vi "LVClass_HasoEngine Set Preferences Multi Aperture.vi"(0 "HasoEngine in":refnum<class "HasoEngine.lvclass">, 5 "Start sub-aperture Array":T1[](array[typedef]), 7 "Pupil average":dbl=0.5 min=0.0 max=1.0, 9 "AutoStartSub-aperture":bool, 11 "error in (no error)":errorcluster) -> (4 "HasoEngine out":refnum<class "HasoEngine.lvclass">, 15 "error out":errorcluster)   [LabVIEW 2020, in "HasoEngine.lvclass"]
doc: "HasoSlopes computation preferences setter.\n\n--------------------------------------------------------------------------------\n\n<B>HasoEngineIn </B> : HasoEngine object.\n<B>HasoEngineOut </B> : HasoEngine object.\n<B>start_subpupil array </B> : Array of sub pupil coordinates to define multi aperture slopes computing option (index coordinates relative to the top-left corner of the pupil).\n<B>denoising_strength </B> : Sensitivity of spot detection on summed images (between 0 and 1).\n<B>auto start activation </B> : Activation of the auto start subpupil detection in case specified start subpupil is not found\n<B>ErrorIn </B> : Error\n<B>ErrorOut </B> : Error\n\n--------------------------------------------------------------------------------"
uses:
  HasoEngine.lvclass
  Point2D.ctl
  HasoEngine.lvclass/HasoEngine.ctl
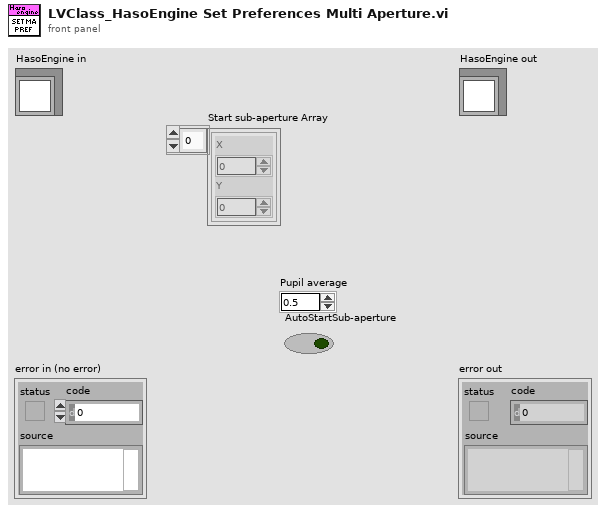
[diagram p1: front panel]
types:
  T1 = typedef "Point2D.ctl" = cluster{"X":u32, "Y":u32}
  T2 = typedef "ClassID.ctl" = i64
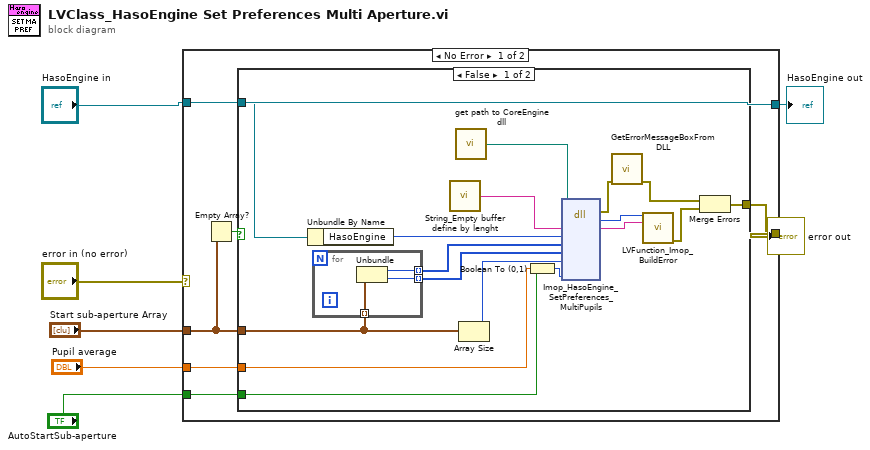
[diagram p0: block diagram]
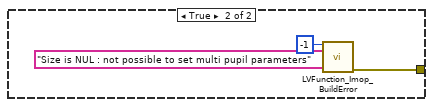
[diagram p2: hidden frame]
diagram:
  n1 = case shown="No Error" "error in (no error)" {
    selector: "error in (no error)" -> [_ w37]
    tunnel: "HasoEngine in" -> [w13 w38]
    tunnel: [w13 w38] -> w4
    tunnel: [w12 w37] -> w5
    tunnel: "AutoStartSub-aperture" -> [w11 _]
    tunnel: "Pupil average" -> [w10 _]
    tunnel: "Start sub-aperture Array" -> [w8 _]
    frame No Error {
      n2 = Empty Array?(array=w8) -> (empty?=w9:bool)
      n3 = case shown="False" w9 {
        tunnel: w13 -> [w25 _]
        tunnel: [w21 w36] -> w12
        tunnel: w11 -> [w19 _]
        tunnel: w10 -> [w18 _]
        tunnel: w8 -> [w16 _]
        frame False {
          n4 = Unbundle By Name(w25) -> ("HasoEngine"=w24:T2)
          n5 = for {
            tunnel: w16 -> [w33] mode=indexing
            tunnel: [w32] -> w15 mode=indexing
            tunnel: [w31] -> w14 mode=indexing
            n6 = Unbundle(w33) -> ("X"=w32:u32, "Y"=w31:u32)
          }
          n7 = call "String_Empty buffer define by lenght.vi"() -> ("Empty buffer"=w28:string)  [unwired: 1 in]
          n8 = call "get path to CoreEngine dll.vi"() -> ("path to wavekit library"=w27:path)  [unwired: 14 in, 1 out]
          n9 = Array Size(array=w16) -> (size(s)=w17:i32)
          n10 = Boolean To (0,1)(Boolean=w19) -> (0, 1=w20:i16)
          n11 = dll-call lib="D:/2_trunk/Soft_haso/ImOpCoreEngine4_LV2011/DLLs/ImopEngine4_vc100.dll" fn="Imop_HasoEngine_SetPreferences_MultiPupils"(path in=w27, "message"=w28, "objet"=w24, "ArrayOfStartSubPupil_X"=w15, "ArrayOfStartSubPupil_Y"=w14, "size"=w17, "pupil_average"=w18, "AutoStartSub-aperture"=w20) -> (error out=w26:errorcluster, "return type"=w29:i32, "message"=w30:string)  [unwired: 8 in, 1 out]
          n12 = call "GetErrorMessageBoxFromDLL.vi"("error IN"=w26) -> ("error OUT"=w23:errorcluster)  [unwired: 10 in]
          n13 = call "LVFunction_Imop_BuildError.vi"("code"=w29, "String to Prepend to source (\"\")"=w30) -> ("error out"=w22:errorcluster)  [unwired: 13 in]
          n14 = Merge Errors(w23, w22) -> (w21:errorcluster)
        }
        frame True {
          n15 = call "LVFunction_Imop_BuildError.vi"("code"=-1, "String to Prepend to source (\"\")"="Size is NUL : not possible to set multi pupil parameters" ("String to Prepend to source (\"\")")) -> ("error out"=w36:errorcluster)  [unwired: 13 in]
        }
      }
    }
    frame Error {
    }
  }
  "error out" <- w5
  "HasoEngine out" <- w4
